vi "Simulate Temperature Acquisition.vi"() -> (3 "temperature":dbl)   [LabVIEW 2023]
doc: "Produces simulated temperature values."
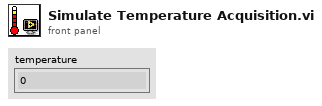
[diagram p1: front panel]
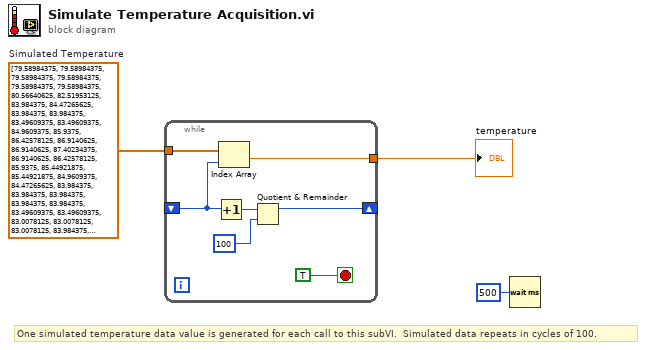
[diagram p0: block diagram]
diagram:
  w3 = dbl[] [79.58984375, 79.58984375, 79.58984375, 79.58984375, 79.58984375, 79.58984375, 80.56640625, 82.51953125, 83.984375, 84.47265625, 83.984375, 83.984375, 83.49609375, 83.49609375, 84.9609375, 85.9375, 86.42578125, 86.9140625, 86.9140625, 87.40234375, 86.9140625, 86.42578125, 85.9375, 85.44921875, 85.44921875, 84.9609375, 84.47265625, 83.984375, 83.984375, 83.984375, 83.984375, 83.984375, 83.49609375, 83.49609375, 83.0078125, 83.0078125, 83.0078125, 83.984375, 84.47265625, 84.9609375, 85.44921875, 86.42578125, 86.9140625, 86.9140625, 86.9140625, 86.42578125, 85.9375, 85.44921875, 85.9375, 86.9140625, 87.40234375, 87.890625, 87.40234375, 86.9140625, 86.9140625, 85.9375, 85.9375, 85.9375, 84.9609375, 84.9609375, 84.9609375, 84.47265625, 84.47265625, 85.44921875, 85.9375, 86.9140625, 86.9140625, 86.42578125, 85.9375, 85.44921875, 85.44921875, 84.9609375, 84.9609375, 84.47265625, 84.47265625, 83.984375, 83.984375, 83.49609375, 83.49609375, 83.0078125, 83.0078125, 83.0078125, 83.0078125, 83.0078125, 83.0078125, 83.0078125, 82.51953125, 81.0546875, 81.54296875, 82.51953125, 83.0078125, 82.51953125, 82.03125, 82.03125, 82.03125, 82.03125, 81.54296875, 81.54296875, 81.54296875, 81.54296875]  # Simulated Temperature
  # "One simulated temperature data value is generated for each call to this subVI.  Simulated data repeats in cycles of 100."
  n1 = while {
    tunnel: w3 -> [w5]
    tunnel: [w6] -> w1
    shift-left: _ -> [w10]
    shift-right: [w7] -> _
    stop <- TRUE stop-if-true
    n2 = Increment(x=w10) -> (x+1=w9:i32)
    n3 = Index Array(array=w5, index=w10) -> (element=w6:dbl)
    n4 = Quotient & Remainder(x=w9, y=100) -> (x-y*floor(x/y)=w7:i32)  [unwired: 1 out]
  }
  "temperature" <- w1
  n5 = Wait (ms)(milliseconds to wait=u32 500) -> ()  [unwired: 1 out]
